vi "XY_MoveToPosition_CT.vi"(10 "Positon (X / Y)":i32[](array[numeric])) -> (2 "Command":string)   [LabVIEW 2017]
uses:
  sobot structures/SoBot_CommandTypes.ctl
  sobot structures/XY_Commands.ctl
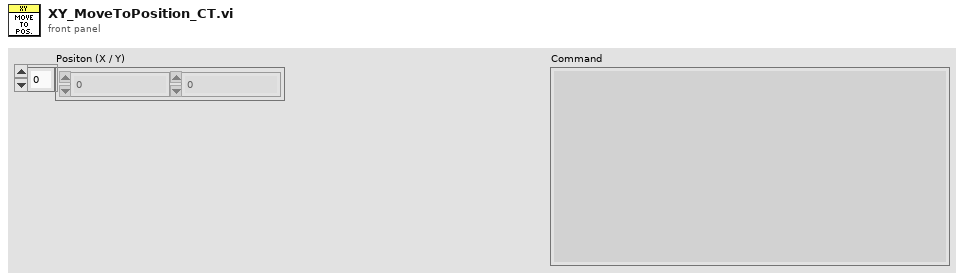
[diagram p1: front panel]
types:
  T1 = typedef "XY_Commands.ctl" = enum16{"XY_Initialize", "XY_MoveToPosition", "XY_MarkTarget", "XY_LockMotors", "XY_UnlockMotors"}
  T2 = typedef "SoBot_CommandTypes.ctl" = enum16{"General_Command", "XY_Command", "Z_Command", "Plattform_Command"}
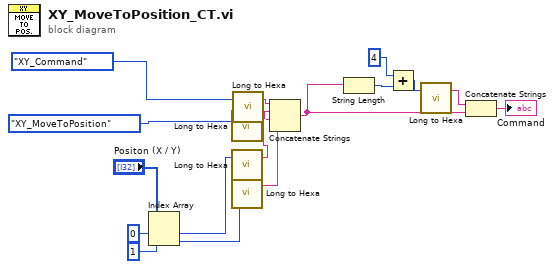
[diagram p0: block diagram]
diagram:
  n1 = Index Array(array="Positon (X / Y)", index #1=0 ("index"), index #2=1 ("index")) -> (element #1=w4:i32, element #2=w3:i32)
  n2 = call "Long to Hexa.vi"("Long"=XY_Commands."XY_MoveToPosition" ("XY_Command")) -> ("Hexa"=w16:string)  [unwired: 2 in]
  n3 = call "Long to Hexa.vi"("Long"=w4) -> ("Hexa"=w7:string)  [unwired: 2 in]
  n4 = call "Long to Hexa.vi"("Long"=w3) -> ("Hexa"=w6:string)  [unwired: 2 in]
  n5 = call "Long to Hexa.vi"("Long"=SoBot_CommandTypes."XY_Command" ("SoBot_CommandTypes")) -> ("Hexa"=w17:string)  [unwired: 2 in]
  n6 = Concatenate Strings(w17, w16, w7, w6) -> (w11:string)
  n7 = String Length(string=w11) -> (length=w15:i32)
  n8 = Add(x=4, y=w15) -> (x+y=w13:i32)
  n9 = call "Long to Hexa.vi"("Long"=w13) -> ("Hexa"=w12:string)  [unwired: 2 in]
  n10 = Concatenate Strings(w12, w11) -> (→"Command":string)
